vi "Get Command Infos.vi"(8 "error in (no error)":errorcluster, 11 "Xbox Controller in":refnum<class "Xbox Controller.lvclass">) -> (0 "error out":errorcluster, 3 "Xbox Controller out":refnum<class "Xbox Controller.lvclass">, 4 "Direction info out":string, 6 "Boost info out":string)   [LabVIEW 2021, in "Xbox Controller.lvclass"]
doc: "MIT Licence\nCopyright (c) 2024 David Grollier"
uses:
  Xbox Controller.lvclass
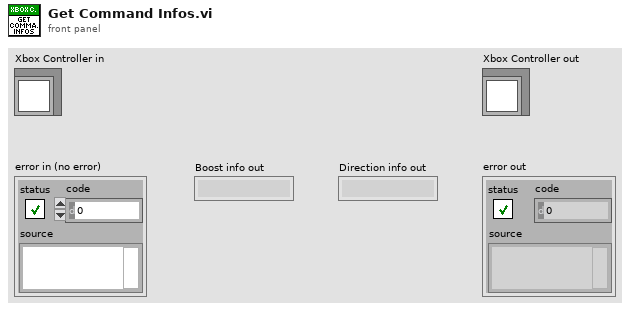
[diagram p1: front panel]
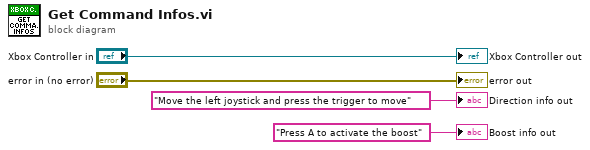
[diagram p0: block diagram]
diagram:
  "error out" <- "error in (no error)"
  "Xbox Controller out" <- "Xbox Controller in"
  "Direction info out" <- "Move the left joystick and press the trigger to move" ("Direction info out")
  "Boost info out" <- "Press A to activate the boost" ("Boost info out")
